vi "Config.vi"(8 "error in (no error)":errorcluster, 9 "Path":path, 10 "Section":string, 11 "Sim Camera Driver in":refnum<class "Sim Camera Driver.lvclass">) -> (0 "error out":errorcluster, 3 "Sim Camera Driver out":refnum<class "Sim Camera Driver.lvclass">)   [LabVIEW 2022 SP3, in "Sim Camera Driver.lvclass"]
uses:
  Sim Camera Driver.lvclass
  Sim Camera Driver.lvclass/Sim Camera Driver.ctl
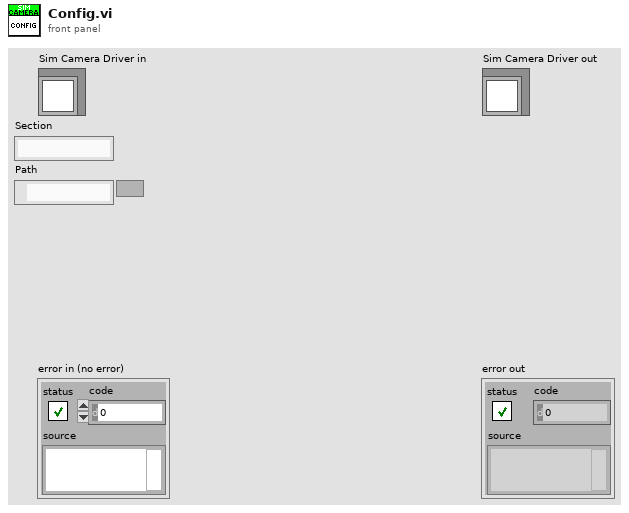
[diagram p1: front panel]
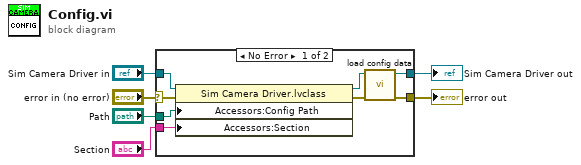
[diagram p0: block diagram]
diagram:
  n1 = case shown="No Error" "error in (no error)" {
    selector: "error in (no error)" -> [w9 w16]
    tunnel: [w7 w16] -> w5
    tunnel: [w10 w15] -> w3
    tunnel: "Sim Camera Driver in" -> [w14 w15]
    tunnel: "Path" -> [w13 _]
    tunnel: "Section" -> [w12 _]
    frame No Error {
      n2 = property class="Sim Camera Driver.lvclass"(reference=w14, error in=w9, "Accessors:Config Path"=w13, "Accessors:Section"=w12) -> (reference out=w11:refnum<class "Sim Camera Driver.lvclass">, error out=w8:errorcluster)
      n3 = call-dynamic "load config data.vi"("error in (no error)"=w8, "Sim Camera Driver in"=w11) -> ("error out"=w7:errorcluster, "Sim Camera Driver out"=w10:refnum<class "Sim Camera Driver.lvclass">)  [unwired: 8 in]
    }
    frame Error {
    }
  }
  "error out" <- w5
  "Sim Camera Driver out" <- w3
